vi "DAQmx Create Channel (TEDS-AI-Bridge).vi"(0 "task in":refnum<k21>, 1 "maximum value":dbl=0.002 format="%.3f", 2 "minimum value":dbl=-0.002 format="%.3f", 5 "physical channels":tag, 7 "name to assign":string, 9 "units":i32(ring)=12516 items=["From TEDS"=12516, "From Custom Scale"=10065], 11 "error in":errorcluster, 12 "custom scale name":tag, 13 "voltage excitation source":i32(ring)=10200 items=["Internal"=10200, "External"=10167], 14 "voltage excitation value":dbl=2.5) -> (4 "task out":refnum<k21>, 15 "error out":errorcluster)   [LabVIEW 2018]
doc: "Creates channel(s) that measure a Wheatstone bridge. You must configure the physical channel(s) with TEDS information to use this VI. Use this instance with bridge-based sensors that measure phenomena other than strain, force, pressure, or torque, or that scale data to physical units NI-DAQmx does not support."
uses:
  nilvaiu.dll
panel:
  # "input limits"
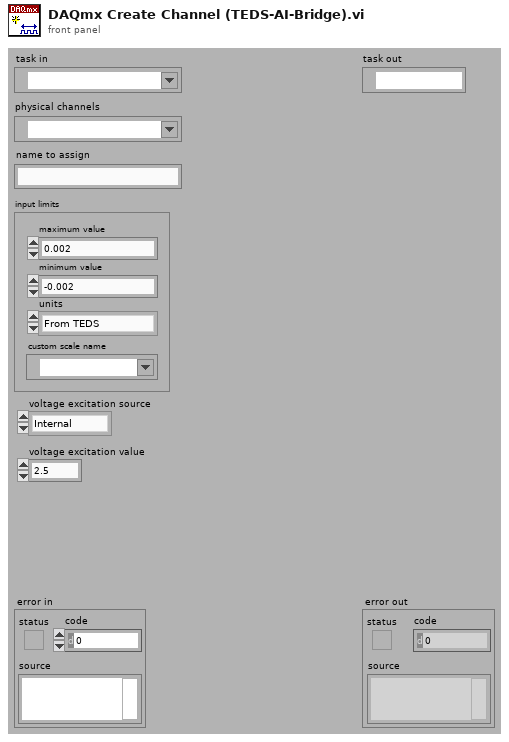
[diagram p1: front panel]
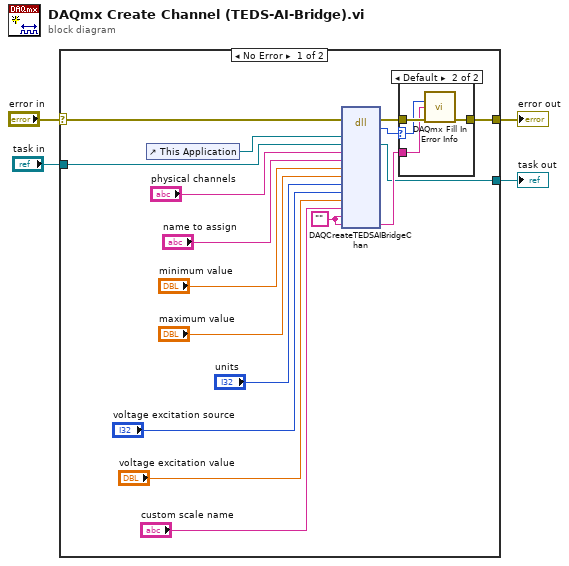
[diagram p0: block diagram]
diagram:
  n1 = case shown="No Error" "error in" {
    selector: "error in" -> [w10 w27]
    tunnel: [w13 w27] -> w4
    tunnel: "task in" -> [w15 w28]
    tunnel: [w14 w28] -> w1
    frame No Error {
      w5 = ""
      n2 = control-ref of="This Application"() -> (w21:refnum<vi>)
      n3 = dll-call lib="nilvaiu.*" fn="DAQCreateTEDSAIBridgeChan"(error in=w10, "lvAppRef"=w21, "refObjPtr"=w15, "physicalChannelName"="physical channels", "channelNameIn"="name to assign", "minVal"="minimum value", "maxVal"="maximum value", "units"="units", "voltageExcitSource"="voltage excitation source", "voltageExcitVal"="voltage excitation value", "customScaleName"="custom scale name", "channelNamesOut"=w5, "extendedErrorInfo"=w5) -> (error out=w20:errorcluster, "return type"=w19:i32, "refObjPtr"=w14:refnum<k21>, "extendedErrorInfo"=w18:string)  [unwired: 12 in, 1 out]
      n4 = case shown="Default" w19 {
        selector: w19 -> [_ w24]
        tunnel: w20 -> [w22 w26]
        tunnel: [w22 w25] -> w13
        tunnel: w18 -> [_ w23]
        frame 0 {
        }
        frame Default {
          n5 = call "DAQmx Fill In Error Info.vi"("status code"=w24, "extended error info"=w23, "error in"=w26) -> ("error out"=w25:errorcluster)  [unwired: 1 in, 11 out]
        }
      }
    }
    frame Error {
    }
  }
  "error out" <- w4
  "task out" <- w1
